vi "tcpServerCallBack.vi"(8 "error in (no error)":errorcluster, 11 "TcpServer in":refnum<class "TcpServer.lvclass">) -> (0 "error out":errorcluster, 3 "TcpServer out":refnum<class "TcpServer.lvclass">)   [LabVIEW 2018, in "TcpServer.lvclass"]
doc: "Receive the incomming json command from TCP Client and process it, and send the results as an user event to the LabVIEW Component."
uses:
  TcpServer.lvclass
  TcpServer.lvclass/TcpServer.ctl
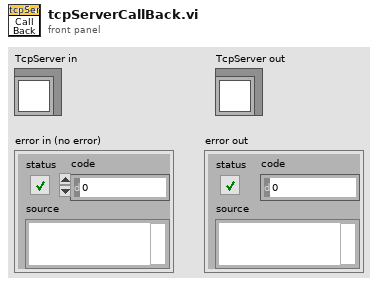
[diagram p1: front panel]
types:
  T1 = typedef "TcpServer.lvclass/packetConnIDTypeDef.ctl" = cluster{"packet":string, "tcpConnectionID":refnum<k5>, "firstPacket":bool, "firstConnection":bool}
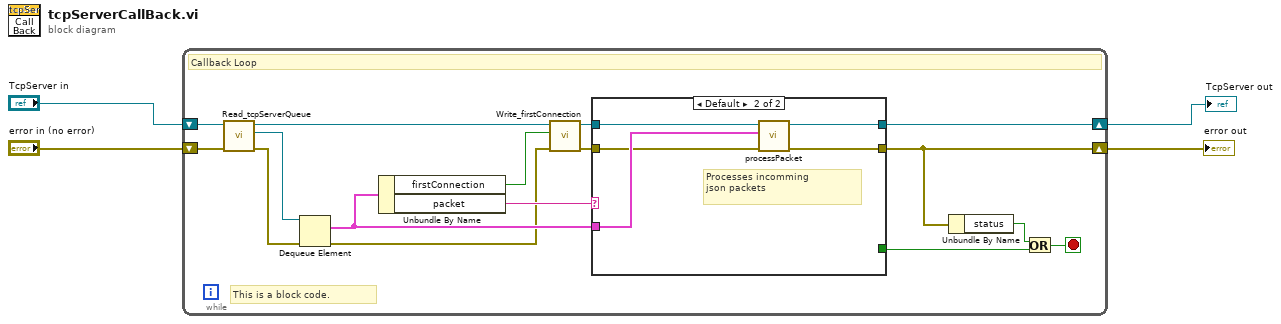
[diagram p0: block diagram]
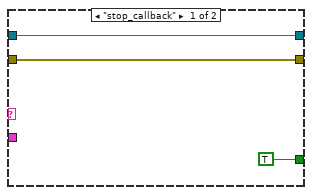
[diagram p2: hidden frame]
diagram:
  n1 = while {
    shift-right: [w15] -> w4
    shift-left: "error in (no error)" -> [w18]
    shift-right: [w12] -> w1
    shift-left: "TcpServer in" -> [w19]
    stop <- w17 stop-if-true
    # "This is a block code."
    # "Callback Loop"
    n2 = call "Read_tcpServerQueue.vi"("error in (no error)"=w18, "tcpServer in"=w19) -> ("error out"=w9:errorcluster, "tcpServerQueue"=w20:refnum<queue>, "tcpServer out"=w11:refnum<class "TcpServer.lvclass">)  [unwired: 7 in]
    n3 = Dequeue Element(queue=w20, error in (no error)=w9) -> (element=w10:T1, error out=w6:errorcluster)  [unwired: 1 in, 2 out]
    n4 = Unbundle By Name(w10) -> ("firstConnection"=w7:bool, "packet"=w13:string)
    n5 = call "Write_firstConnection.vi"("error in (no error)"=w6, "firstConnection"=w7, "TcpServer in"=w11) -> ("error out"=w5:errorcluster, "TcpServer out"=w8:refnum<class "TcpServer.lvclass">)  [unwired: 7 in]
    n6 = case shown="Default" w13 {
      tunnel: w8 -> [w22 w28]
      tunnel: [TRUE _] -> w16
      tunnel: [w21 w27] -> w15
      tunnel: w10 -> [_ w26]
      tunnel: [w22 w25] -> w12
      tunnel: w5 -> [w21 w24]
      frame "stop_callback" {
      }
      frame Default {
        # "Processes incomming\njson packets"
        n7 = call "processPacket.vi"("error in (no error)"=w24, "packetConnID"=w26, "tcpServer in"=w28) -> ("error out"=w27:errorcluster, "tcpServer out"=w25:refnum<class "TcpServer.lvclass">)  [unwired: 7 in]
      }
    }
    n8 = Unbundle By Name(w15) -> ("status"=w14:bool)
    n9 = Or(x=w14, y=w16) -> (x .or. y?=w17:bool)
  }
  "error out" <- w4
  "TcpServer out" <- w1
